vi "Untitled 6.vi"() -> ()   [LabVIEW 2014]
uses:
  <vilib>/Instr/_visa.llb/VISA Configure Serial Port (Instr).vi
panel:
  out "MCode get":string
  in  "Send":bool
  in  "Gcode":string
  in  "String":string
  out "error out":errorcluster
  in  "stop":bool
  out "concatenated string":string
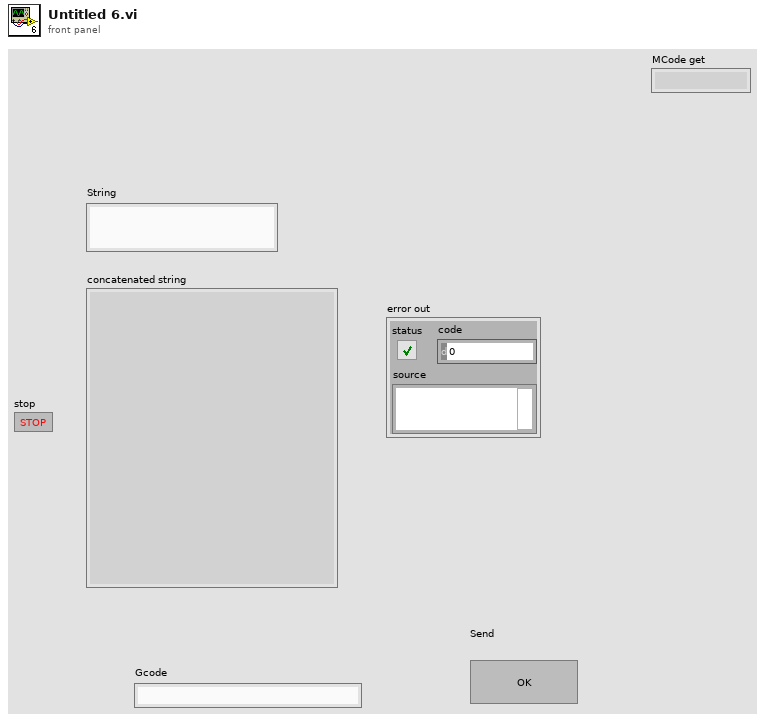
[diagram p1: front panel]
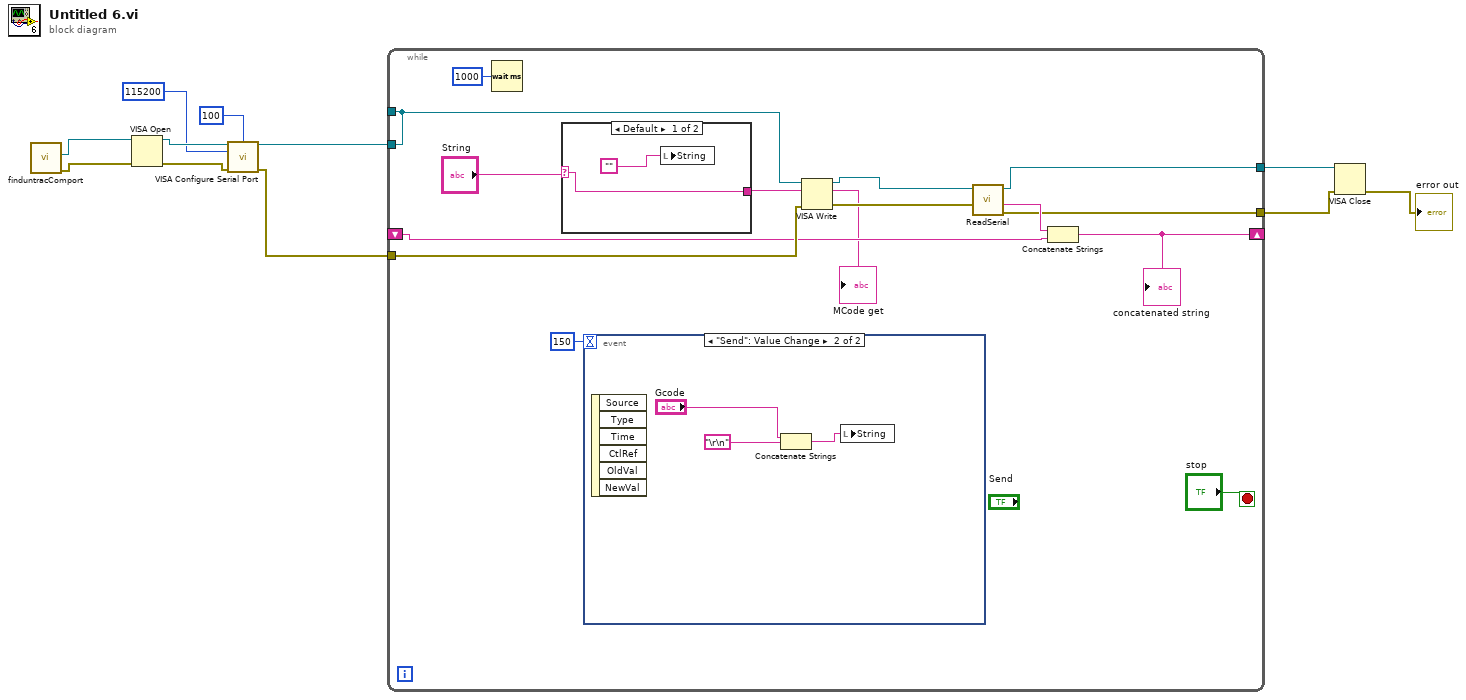
[diagram p0: block diagram]
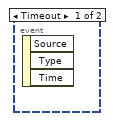
[diagram p2: hidden frame]
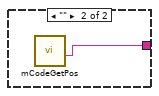
[diagram p3: hidden frame]
diagram:
  n1 = call "finduntracComport.vi"() -> ("OUT COM"=w11:refnum<visa-resource-name>, "error out"=w10:errorcluster)  [unwired: 9 in]
  n2 = VISA Open(error in (no error)=w10, VISA resource name=w11) -> (VISA resource name=w6:refnum<visa-resource-name>, error out=w3:errorcluster)  [unwired: 3 in]
  n3 = call-poly "VISA Configure Serial Port"("VISA resource name"=w6, "termination char\n(0xA = '\\n' = LF)"=u8 100 ("termination char\n(0xA = '\\n' = LF)"), "baud rate (9600)"=u32 115200, "error in (no error)"=w3) -> ("VISA resource name out"=w5:refnum<visa-resource-name>, "error out"=w4:errorcluster)  [unwired: 10 in]
  n4 = while {
    tunnel: w4 -> [w25]
    tunnel: [w12] -> _
    shift-right: [w21] -> _
    shift-left: _ -> [w20]
    tunnel: [w17] -> w8
    tunnel: [w16] -> w7
    tunnel: w5 -> [w12]
    stop <- "stop" stop-if-true
    n5 = Wait (ms)(milliseconds to wait=u32 1000) -> ()  [unwired: 1 out]
    n6 = case shown="Default" "String" {
      selector: "String" -> [w29 _]
      tunnel: [w29 w31] -> w13
      frame Default {
        n7 = local write "String"("") -> ()
      }
      frame "" {
        n8 = call "mCodeGetPos.vi"() -> ("MCode get"=w31:string)  [unwired: 11 in]
      }
    }
    "MCode get" <- w13
    n9 = event shown="[1] \"Send\": Value Change" {
      selector: _ -> [_ _]
      dyn-events: _ -> [_ _]
      timeout: 150 -> [_ _]
      event Timeout {
        n10 = event-data() -> ()  [unwired: 1 in, 3 out]
      }
      event "Send": Value Change {
        n11 = event-data() -> ()  [unwired: 1 in, 6 out]
        n12 = Concatenate Strings("Gcode", "\r\n") -> (w27:string)
        n13 = local write "String"(w27) -> ()
      }
    }
    n14 = VISA Write(VISA resource name=w12, write buffer=w13, error in (no error)=w25) -> (VISA resource name out=w24:refnum<visa-resource-name>, error out=w23:errorcluster)  [unwired: 1 out]
    n15 = call "ReadSerial.vi"("error in (no error)"=w23, "VISA IN"=w24) -> ("error out"=w17:errorcluster, "bufferOut"=w22:string, "VISA  OUT"=w16:refnum<visa-resource-name>)  [unwired: 7 in]
    n16 = Concatenate Strings(w22, w20) -> (w21:string)
    "concatenated string" <- w21
  }
  n17 = VISA Close(VISA resource name=w7, error in (no error)=w8) -> (error out=→"error out":errorcluster)
